vi "Add to Project.vi"(8 "error in (no error)":errorcluster, 11 "Abstract Message Rescripter in":refnum<class "Abstract Message Rescripter.lvclass">) -> (0 "error out":errorcluster, 3 "Abstract Message Rescripter out":refnum<class "Abstract Message Rescripter.lvclass">)   [LabVIEW 2020, in "Message Rescripter.lvlib" / "Abstract Message Rescripter.lvclass"]
uses:
  Abstract Message Rescripter.lvclass
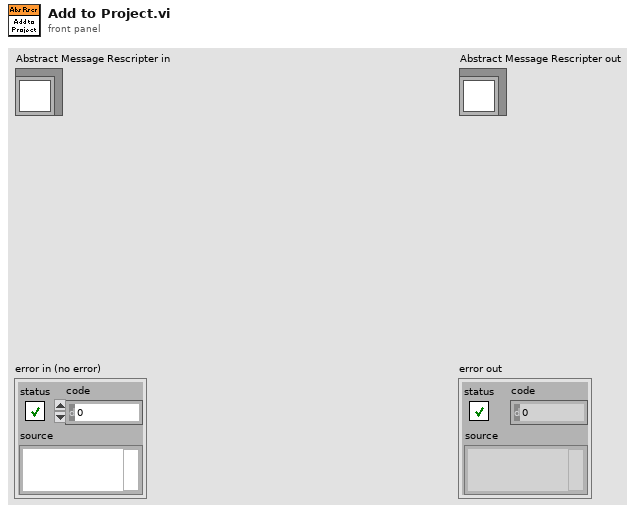
[diagram p1: front panel]
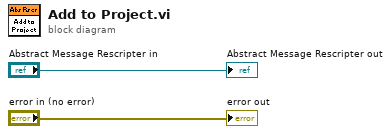
[diagram p0: block diagram]
diagram:
  "error out" <- "error in (no error)"
  "Abstract Message Rescripter out" <- "Abstract Message Rescripter in"
